vi "filter_average_by_target.vi"(6 "Target id to track":string, 7 "Targets":T1(array[cluster])) -> (1 "Average Velocity":sgl, 2 "Average Range":sgl, 3 "Average AoA":sgl)   [LabVIEW 2019, in "Lib_Simx.lvlib"]
doc: "Filter targets and calculate average for AoA, range and velocity for the specified target id when there are multiple targets with the same target id."
uses:
  Lib_Simx.lvlib
panel:
  out "Target found at  Index":i32[](array[numeric])
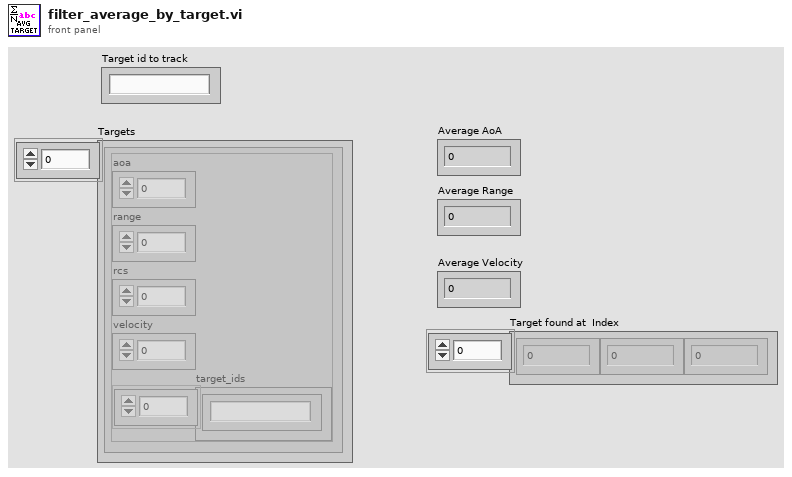
[diagram p1: front panel]
types:
  T1 = cluster{"aoa":sgl, "range":sgl, "rcs":sgl, "velocity":sgl, "target_ids":string[]}[]
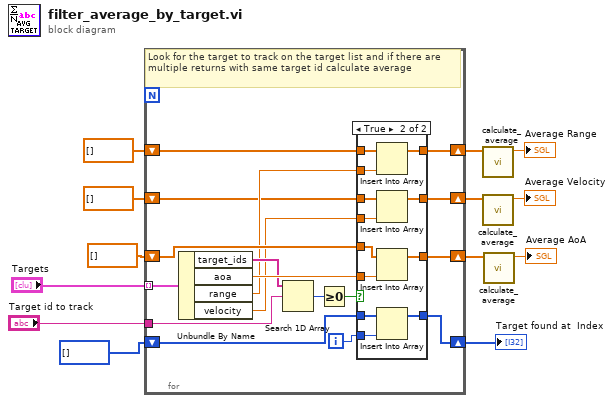
[diagram p0: block diagram]
diagram:
  n1 = for {
    tunnel: "Targets" -> [w30] mode=indexing
    tunnel: "Target id to track" -> [w25]
    shift-right: [w20] -> w5
    shift-left: sgl[] [] -> [w29]
    shift-right: [w22] -> w4
    shift-left: i32[] [] ("Array 2") -> [w23]
    shift-right: [w17] -> w7
    shift-left: sgl[] [] -> [w19]
    shift-right: [w14] -> w8
    shift-left: sgl[] [] -> [w16]
    i -> [w21]
    # "Look for the target to track on the target list and if there are multiple returns with same target id calculate average"
    n2 = Unbundle By Name(w30) -> ("target_ids"=w26:string[], "aoa"=w28:sgl, "range"=w18:sgl, "velocity"=w15:sgl)
    n3 = Search 1D Array(1D array=w26, element=w25) -> (index of element=w27:i32)  [unwired: 1 in]
    n4 = Greater Or Equal To 0?(x=w27) -> (x >= 0?=w24:bool)
    n5 = case shown="True" w24 {
      tunnel: w28 -> [_ w44]
      tunnel: w29 -> [w34 w46]
      tunnel: [w34 w45] -> w20
      tunnel: w23 -> [w33 w43]
      tunnel: [w33 w42] -> w22
      tunnel: w21 -> [_ w41]
      tunnel: w19 -> [w32 w40]
      tunnel: w18 -> [_ w39]
      tunnel: [w32 w38] -> w17
      tunnel: w16 -> [w31 w37]
      tunnel: w15 -> [_ w36]
      tunnel: [w31 w35] -> w14
      frame False {
      }
      frame True {
        n6 = Insert Into Array(array=w40, new element=w39) -> (w38:sgl[])  [unwired: 1 in]
        n7 = Insert Into Array(array=w37, new element=w36) -> (w35:sgl[])  [unwired: 1 in]
        n8 = Insert Into Array(array=w46, new element=w44) -> (w45:sgl[])  [unwired: 1 in]
        n9 = Insert Into Array(array=w43, new element=w41) -> (w42:i32[])  [unwired: 1 in]
      }
    }
  }
  "Target found at  Index" <- w4
  n10 = call "calculate_average.vi"("Values to average"=w7) -> ("Average"=→"Average Range":sgl)  [unwired: 5 in, 1 out]
  n11 = call "calculate_average.vi"("Values to average"=w8) -> ("Average"=→"Average Velocity":sgl)  [unwired: 5 in, 1 out]
  n12 = call "calculate_average.vi"("Values to average"=w5) -> ("Average"=→"Average AoA":sgl)  [unwired: 5 in, 1 out]
